vi "Anritsu VNA Read Status Bit.vi"(7 "Anritsu VNA":T1, 8 "error in (no error)":errorcluster, 10 "STB Only? (f: Read registers)":bool, 11 "VISA Resource Name":refnum<visa-resource-name>) -> (0 "error out":errorcluster, 2 "OPC Bit":bool, 3 "dup VISA Resource Name":refnum<visa-resource-name>)   [LabVIEW 2011]
doc: "This VI for the HP8753B Network Analyzer reads the status byte and the two event status registers. The two status registers are read out as regular output and will therefore clear anything already in the output queue."
uses:
  TypeDefs/Anritsu VNA Instrument Info.ctl
panel:
  out "Extended Event Status Register":bool[](array[boolean])
  out "Event Status Register":bool[](array[boolean])
  out "Status Byte":bool[](array[boolean])
  # "Calibration Complete (CAC)\n\nNot Used\n\nNot Used\n\nSweep Complete (SWC)\n\nNot Used\n\nNot Used\n\nNot Used\n\nNot Used\n\nNew Service Log Entry (NSE)\n\nCollect Buffer Full (CSF)\n\nSweep Changed (SCH)\n\nNot Used\n\nNot Used\n\nNot Used\n\nSequence Complete (SEC)\n\nNot Used"
  # "Operation Complete (OPC)\n\nNot Used\n\nQuery Error (QYE)\n\nDevice Specific Error (DDE)\n\nExecution Error (EXE)\n\nCommand Error (CME)\n\nUser Request (URQ)\n\nPower On (PON)"
  # "Not Used\n\nLimits Event Status (LESB)\n\nNot Used\n\nNot Used\n\nMessage Available (MAV)\n\nStandard Event Status (ESB)\n\nMaster Summary Status (MSS) or Requesting Service (RQS)\n\nExtended Event Status (EESB)"
  # "read status byte only\nread status byte and status registers"
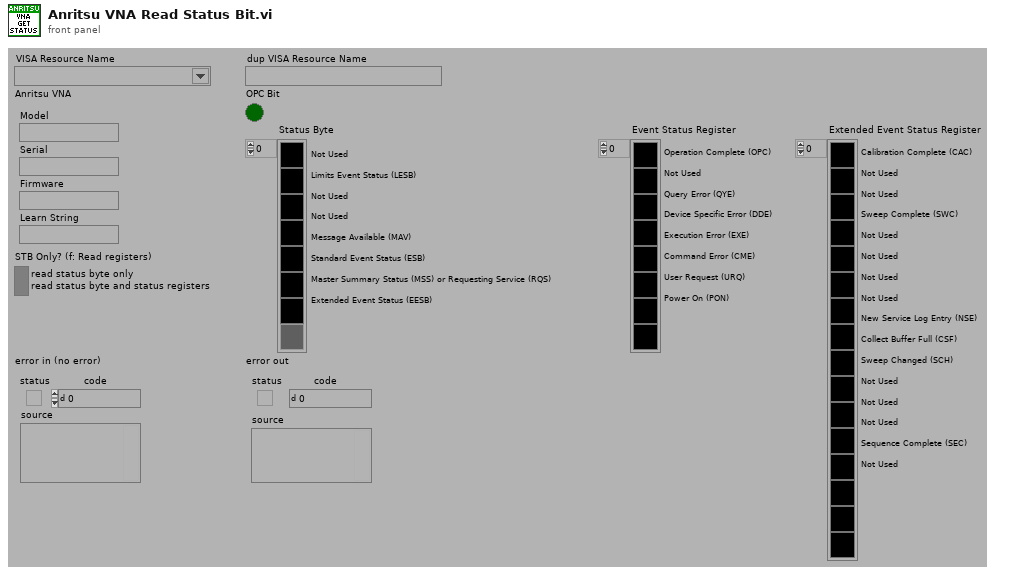
[diagram p1: front panel]
types:
  T1 = typedef "Anritsu VNA Instrument Info.ctl" = cluster{"Model":string, "Serial":string, "Firmware":string, "Learn String":string}
  T2 = typedef "Anritsu VNA Model.ctl" = enum16{"Not Supported", "37XXXX", "MS20XXX", "MS462XX", "MS464XX"}
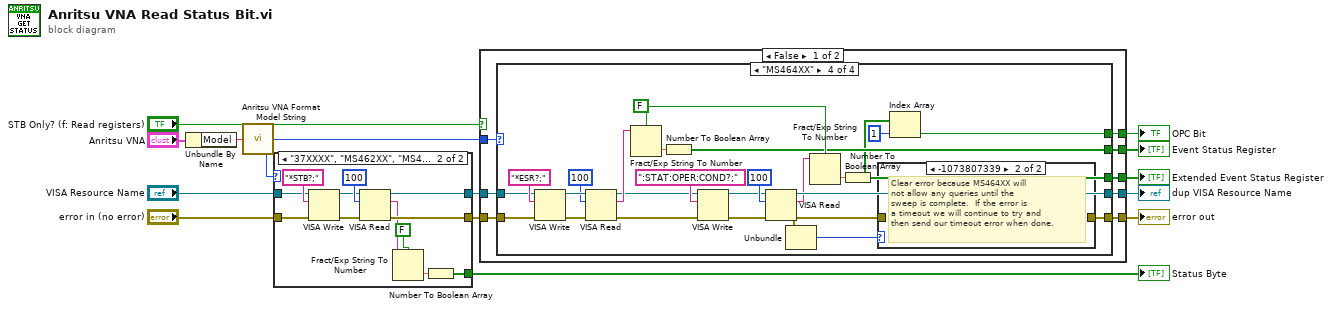
[diagram p0: block diagram]
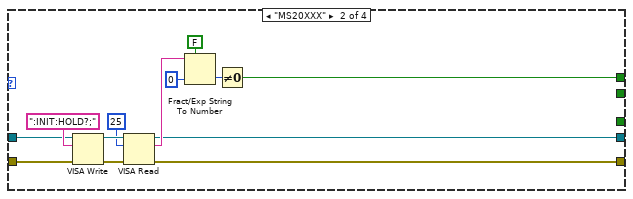
[diagram p4: hidden frame]
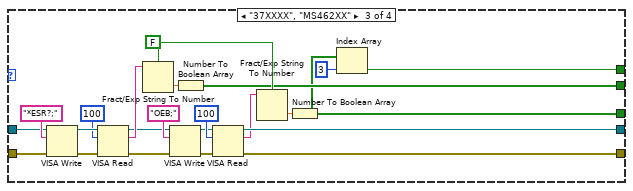
[diagram p5: hidden frame]
diagram:
  n1 = Unbundle By Name("Anritsu VNA") -> ("Model"=w2:string)
  n2 = call "Anritsu VNA Format Model String.vi"("Model"=w2) -> ("Model"=w1:T2)
  n3 = case shown="\"37XXXX\", \"MS462XX\", \"MS464XX\"" w1 {
    tunnel: "error in (no error)" -> [w15 w24]
    tunnel: [w15 w23] -> w6
    tunnel: [w16 w22] -> w5
    tunnel: "VISA Resource Name" -> [w16 w21]
    tunnel: [_ w17] -> w3
    frame "Not Supported", "MS20XXX" {
    }
    frame "37XXXX", "MS462XX", "MS464XX" {
      n4 = VISA Write(VISA resource name=w21, write buffer="*STB?;", error in (no error)=w24) -> (VISA resource name out=w26:refnum<visa-resource-name>, error out=w25:errorcluster)  [unwired: 1 out]
      n5 = VISA Read(VISA resource name=w26, byte count=u32 100, error in (no error)=w25) -> (VISA resource name out=w22:refnum<visa-resource-name>, read buffer=w18:string, error out=w23:errorcluster)  [unwired: 1 out]
      n6 = Fract/Exp String To Number(use system decimal point (T)=FALSE, string=w18) -> (number=w20:dbl)  [unwired: 3 out]
      n7 = Number To Boolean Array(number=w20) -> (Boolean array=w17:bool[])
    }
  }
  "Status Byte" <- w3
  n8 = case shown="False" "STB Only? (f: Read registers)" {
    tunnel: [w36 w102] -> w14
    tunnel: [w35 w101] -> w13
    tunnel: [w34 _] -> w12
    tunnel: w6 -> [w33 w102]
    tunnel: w5 -> [w32 w101]
    tunnel: [w31 _] -> w11
    tunnel: [w30 _] -> w9
    tunnel: w1 -> [w29 _]
    frame False {
      n9 = case shown="\"MS464XX\"" w29 {
        tunnel: [w37 w44 w61 w75] -> w36
        tunnel: [w38 w43 w59 w85] -> w35
        tunnel: w32 -> [w38 w42 w70 w95]
        tunnel: w33 -> [w37 w41 w69 w94]
        tunnel: [_ w39 w54 w80] -> w34
        tunnel: [_ _ w56 w82] -> w31
        tunnel: [_ _ w52 w78] -> w30
        frame "Not Supported" {
        }
        frame "MS20XXX" {
          n10 = VISA Write(VISA resource name=w42, write buffer=":INIT:HOLD?;", error in (no error)=w41) -> (VISA resource name out=w50:refnum<visa-resource-name>, error out=w51:errorcluster)  [unwired: 1 out]
          n11 = VISA Read(VISA resource name=w50, byte count=u32 25, error in (no error)=w51) -> (VISA resource name out=w43:refnum<visa-resource-name>, read buffer=w47:string, error out=w44:errorcluster)  [unwired: 1 out]
          n12 = Fract/Exp String To Number(use system decimal point (T)=FALSE, string=w47, default (0 dbl)=0 ("default (0 DBL)")) -> (number=w40:i32)  [unwired: 2 out]
          n13 = Not Equal To 0?(x=w40) -> (x != 0?=w39:bool)
        }
        frame "37XXXX", "MS462XX" {
          w57 = FALSE ("use system decimal point (T)")
          n14 = VISA Write(VISA resource name=w70, write buffer="*ESR?;", error in (no error)=w69) -> (VISA resource name out=w73:refnum<visa-resource-name>, error out=w74:errorcluster)  [unwired: 1 out]
          n15 = VISA Read(VISA resource name=w73, byte count=u32 100, error in (no error)=w74) -> (VISA resource name out=w63:refnum<visa-resource-name>, read buffer=w67:string, error out=w62:errorcluster)  [unwired: 1 out]
          n16 = Fract/Exp String To Number(use system decimal point (T)=w57, string=w67) -> (number=w68:dbl)  [unwired: 3 out]
          n17 = VISA Write(VISA resource name=w63, write buffer="OEB;", error in (no error)=w62) -> (VISA resource name out=w64:refnum<visa-resource-name>, error out=w60:errorcluster)  [unwired: 1 out]
          n18 = Number To Boolean Array(number=w68) -> (Boolean array=w56:bool[])
          n19 = VISA Read(VISA resource name=w64, byte count=u32 100, error in (no error)=w60) -> (VISA resource name out=w59:refnum<visa-resource-name>, read buffer=w58:string, error out=w61:errorcluster)  [unwired: 1 out]
          n20 = Fract/Exp String To Number(use system decimal point (T)=w57, string=w58) -> (number=w55:dbl)  [unwired: 3 out]
          n21 = Number To Boolean Array(number=w55) -> (Boolean array=w52:bool[])
          n22 = Index Array(array=w52, index=3) -> (element=w54:bool)
        }
        frame "MS464XX" {
          w83 = FALSE ("use system decimal point (T)")
          n23 = VISA Write(VISA resource name=w95, write buffer="*ESR?;", error in (no error)=w94) -> (VISA resource name out=w98:refnum<visa-resource-name>, error out=w99:errorcluster)  [unwired: 1 out]
          n24 = VISA Read(VISA resource name=w98, byte count=u32 100, error in (no error)=w99) -> (VISA resource name out=w88:refnum<visa-resource-name>, read buffer=w92:string, error out=w87:errorcluster)  [unwired: 1 out]
          n25 = Fract/Exp String To Number(use system decimal point (T)=w83, string=w92) -> (number=w93:dbl)  [unwired: 3 out]
          n26 = Number To Boolean Array(number=w93) -> (Boolean array=w82:bool[])
          n27 = VISA Write(VISA resource name=w88, write buffer=":STAT:OPER:COND?;", error in (no error)=w87) -> (VISA resource name out=w89:refnum<visa-resource-name>, error out=w86:errorcluster)  [unwired: 1 out]
          n28 = VISA Read(VISA resource name=w89, byte count=u32 100, error in (no error)=w86) -> (VISA resource name out=w85:refnum<visa-resource-name>, read buffer=w84:string, error out=w76:errorcluster)  [unwired: 1 out]
          n29 = Unbundle(w76) -> ("code"=w77:i32)  [unwired: 2 out]
          n30 = Fract/Exp String To Number(use system decimal point (T)=w83, string=w84) -> (number=w81:dbl)  [unwired: 3 out]
          n31 = Number To Boolean Array(number=w81) -> (Boolean array=w78:bool[])
          n32 = case shown="-1073807339" w77 {
            tunnel: w76 -> [w100 _]
            tunnel: [w100 _] -> w75
            frame Default {
            }
            frame -1073807339 {
              # "Clear error because MS464XX will\nnot allow any queries until the\nsweep is complete.  If the error is\na timeout we will continue to try and\nthen send our timeout error when done."
            }
          }
          n33 = Index Array(array=w78, index=1) -> (element=w80:bool)
        }
      }
    }
    frame True {
    }
  }
  "dup VISA Resource Name" <- w13
  "error out" <- w14
  "OPC Bit" <- w12
  "Event Status Register" <- w11
  "Extended Event Status Register" <- w9
